vi "Write Status_Flags_Ref.vi"(8 "error in (no error)":errorcluster, 10 "Status_Flags_Ref":refnum<vi>, 11 "Electronic Load in":refnum<class "Electronic Load.lvclass">) -> (0 "error out":errorcluster, 3 "Electronic Load out":refnum<class "Electronic Load.lvclass">)   [LabVIEW 2019, in "Electronic Load.lvlib" / "Electronic Load.lvclass"]
uses:
  Library/Electronic Load.lvclass
  Custom Controls/Status_Flags.ctl
  Library/Electronic Load.lvclass/Electronic Load.ctl
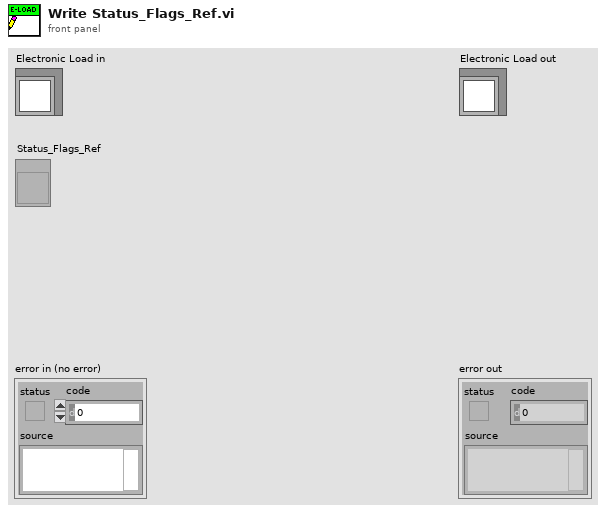
[diagram p1: front panel]
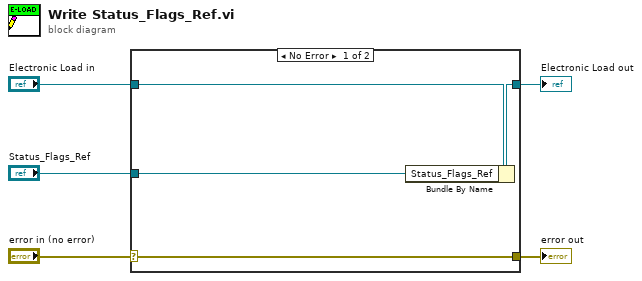
[diagram p0: block diagram]
diagram:
  n1 = case shown="No Error" "error in (no error)" {
    selector: "error in (no error)" -> [w9 w10]
    tunnel: [w9 w10] -> w4
    tunnel: [w7 w11] -> w2
    tunnel: "Electronic Load in" -> [w8 w11]
    tunnel: "Status_Flags_Ref" -> [w6 _]
    frame No Error {
      n2 = Bundle By Name(cluster=w8, "Status_Flags_Ref"=w6) -> (w7:refnum<class "Electronic Load.lvclass">)
    }
    frame Error {
    }
  }
  "error out" <- w4
  "Electronic Load out" <- w2
